vi "begin_ubin.vi"(8 "error in":errorcluster, 11 "file":path) -> (0 "error out":errorcluster, 3 "refnum out":refnum<file>)   [LabVIEW 2012]
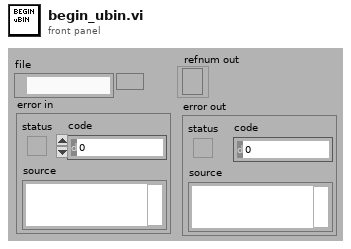
[diagram p1: front panel]
types:
  T1 = enum16{"big-endian, network order", "native, host order", "little-endian"}
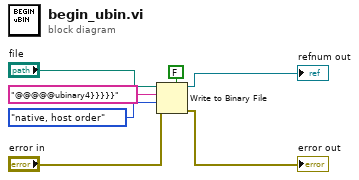
[diagram p0: block diagram]
diagram:
  n1 = Write to Binary File(file (use dialog)="file", data="@@@@@ubinary4}}}}}", error in="error in", 5:FALSE ("prepend array or string size? (T)"), 9:T1."native, host order" ("byte order (0:big-endian, network order)")) -> (refnum out=→"refnum out":refnum<file>, error out=→"error out":errorcluster)  [unwired: 1 in, 1 out]
